vi "Teleop.vi"(10 "Match Info":T1={"Autonomous Elapsed Seconds"=0.0, "TeleOp Elapsed Seconds"=0.0, "Disabled Elapsed Seconds"=0.0, "Visited Autonomous"=FALSE, "Visited TeleOp"=FALSE, "Visited Disabled"=FALSE, "Autonomous Settings"={"Autonomous Style"=enum."Independent", "VI Refnum"=refnum}}, 11 "Call Context":T2) -> ()   [LabVIEW 2023]
doc: "This VI is called for each TeleOp packet received from the DS where the robot is not disabled. It is often used to read from the joysticks and update I/O or to update setpoints for timed control loops. It should complete and return within 20 milliseconds or it may miss DS packets."
uses:
  <vilib>/Rock Robotics/WPI/DriverStation/WPI_DriverStationDerivedRobotMode.ctl
  <vilib>/Rock Robotics/WPI/DriverStation/WPI_DriverStationMatch Info.ctl
  <vilib>/Rock Robotics/Network Tables/NT Read Boolean.vi
  <vilib>/Rock Robotics/WPI/Utilities/WPI_GetSetVariantRefNum.vi
  variavelVelocidades.vi
  <vilib>/Rock Robotics/Network Tables/NT Read Number.vi
  <vilib>/Rock Robotics/WPI/RobotDrive/WPI_RobotDriveArcadeDrive_Standard(NoSaturation).vi
  <vilib>/Rock Robotics/Network Tables/NT Write Boolean.vi
panel:
  out "botaoAtivado?":bool
  out "Sample Slider 0":dbl(slide) scale=0.0..5.0
  out "Sample Boolean 1":bool
  out "Sample Boolean 0":bool
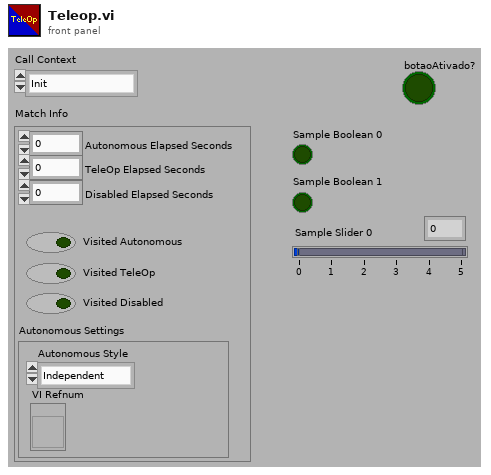
[diagram p1: front panel]
types:
  T1 = typedef "WPI_DriverStationMatch Info.ctl" = cluster{"Autonomous Elapsed Seconds":dbl, "TeleOp Elapsed Seconds":dbl, "Disabled Elapsed Seconds":dbl, "Visited Autonomous":bool, "Visited TeleOp":bool, "Visited Disabled":bool, "Autonomous Settings":cluster{"Autonomous Style":enum16{"Iterative", "Independent"}, "VI Refnum":refnum<vi>}}
  T2 = typedef "WPI_DriverStationDerivedRobotMode.ctl" = enum16{"Init", "Execute", "Stop"}
  T3 = typedef "WPI_JoystickDevRef.ctl" = cluster{"Device":T4}
  T4 = typedef "WPI_JoystickDeviceEnum.ctl" = enum16{"USB 0", "USB 1", "USB 2", "USB 3", "USB 4", "USB 5"}
  T5 = typedef "WPI_RobotDriveDevRef.ctl" = cluster{"DevStatus":errorcluster, "Motors[]":T6[], "Square Inputs":bool, "Max Output":dbl}
  T6 = typedef "WPI_MotorControlDeviceRef.ctl" = cluster{"DeviceStatus":errorcluster, "Type":T7, "PWM":cluster{"PWM Channel":T8, "DeadBand":T9}, "CAN":cluster{"Device Number":u8, "SetOutput VI Ref":variant, "GetOutput VI Ref":variant, "Enable VI Ref":variant, "Disable VI Ref":variant, "Data":variant}, "Invert":bool, "DIO PWM":cluster{"PWM \"Enable\" Channel":T8, "DIOChannel":T10, "PWM Rate":dbl}}
  T7 = typedef "WPI_MotorControlType.ctl" = enum16{"PWM", "CAN", "DIO PWM"}
  T8 = typedef "FPGA_DIOPWMChannel.ctl" = enum8{"PWM 0", "PWM 1", "PWM 2", "PWM 3", "PWM 4", "PWM 5", "PWM 6", "PWM 7", "PWM 8", "PWM 9", "PWM MXP 0", "PWM MXP 1", "PWM MXP 2", "PWM MXP 3", "PWM MXP 4", "PWM MXP 5", "PWM MXP 6", "PWM MXP 7", "PWM MXP 8", "PWM MXP 9", "Invalid"}
  T9 = typedef "WPI_PWMDeadband.ctl" = cluster{"Name":string, "maxPositivePwm":i32, "minPositivePwm":i32, "centerPwm":i32, "maxNegativePwm":i32, "minNegativePwm":i32, "angularRange":u16}
  T10 = typedef "FPGA_DIOChannel.ctl" = enum8{"DIO 0", "DIO 1", "DIO 2", "DIO 3", "DIO 4", "DIO 5", "DIO 6", "DIO 7", "DIO 8", "DIO 9", "DIO MXP 0", "DIO MXP 1", "DIO MXP 2", "DIO MXP 3", "DIO MXP 4", "DIO MXP 5", "DIO MXP 6", "DIO MXP 7", "DIO MXP 8", "DIO MXP 9", "DIO MXP 10", "DIO MXP 11", "DIO MXP 12", "DIO MXP 13", "DIO MXP 14", "DIO MXP 15", "SPI Port CS1", "SPI Port CS2", "SPI Port CS3", "SPI Port MISO", "SPI Port MOSI", "Invalid"}
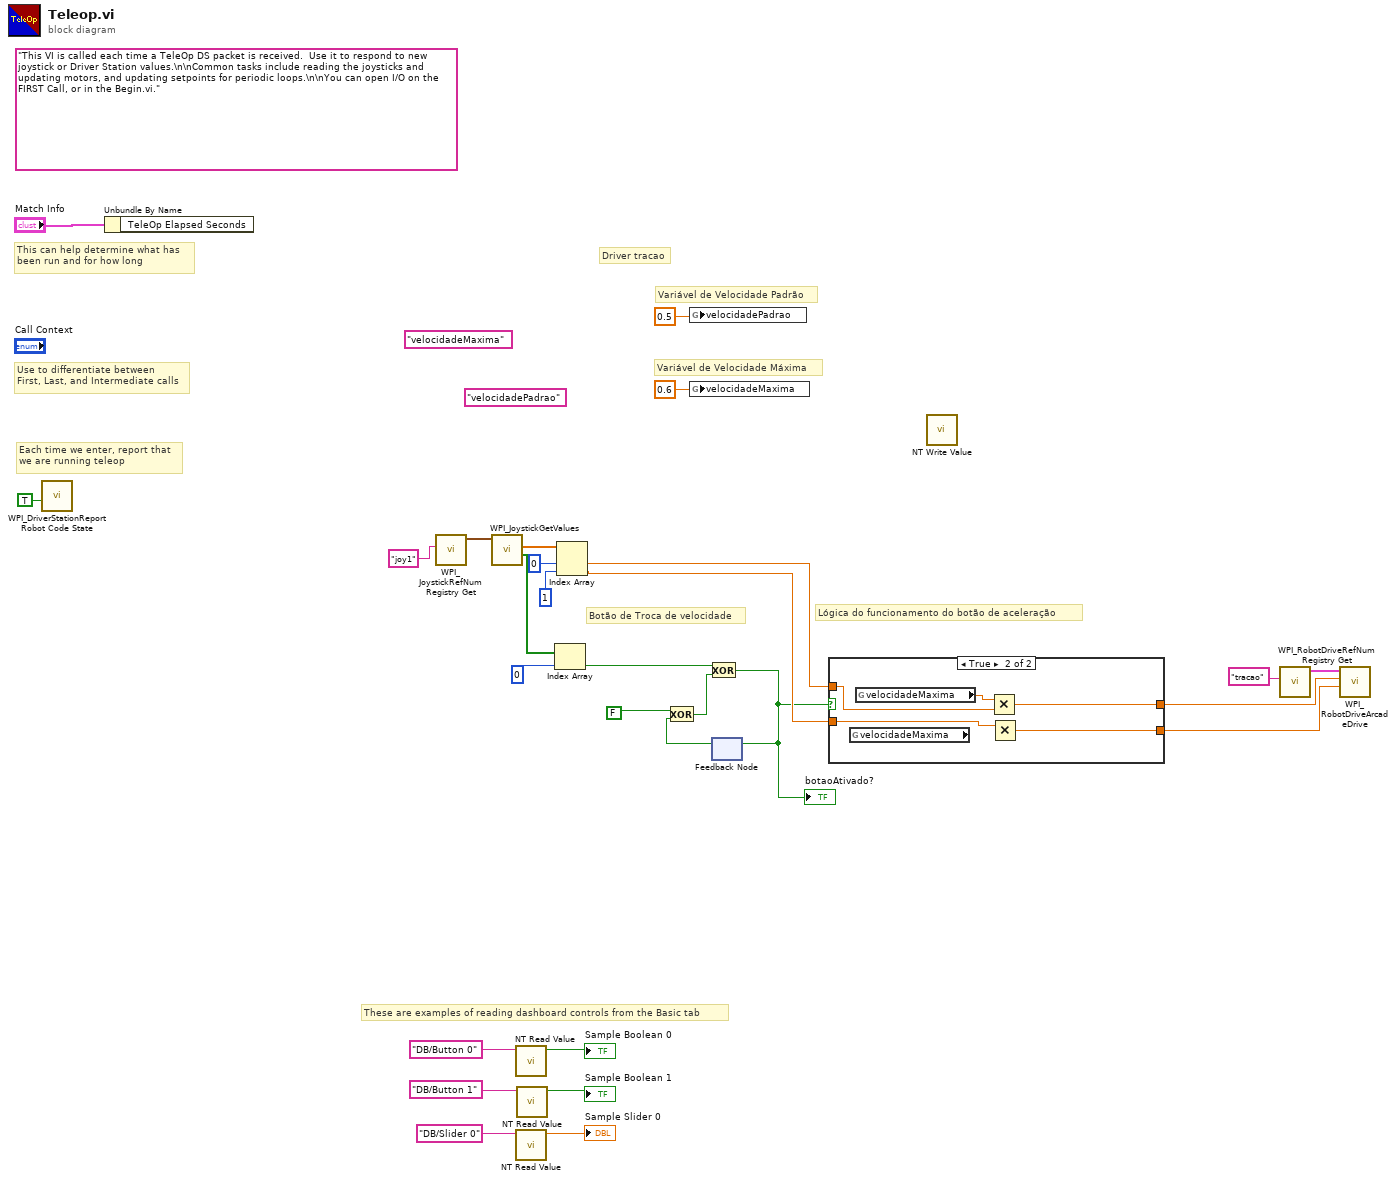
[diagram p0: block diagram]
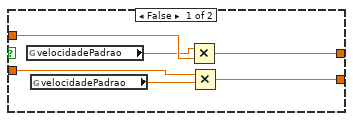
[diagram p2: hidden frame]
diagram:
  (unwired) "velocidadePadrao"
  (unwired) "velocidadeMaxima"
  (unwired) "This VI is called each time a TeleOp DS packet is received.  Use it to respond to new joystick or Driver Station values.\n\nCommon tasks include reading the joysticks and updating motors, and updating setpoints for periodic loops.\n\nYou can open I/O on the FIRST Call, or in the Begin.vi."
  # "Variável de Velocidade Máxima"
  # "Variável de Velocidade Padrão"
  # "Botão de Troca de velocidade"
  # "Lógica do funcionamento do botão de aceleração"
  # "These are examples of reading dashboard controls from the Basic tab"
  # "Each time we enter, report that\nwe are running teleop"
  # "Use to differentiate between\nFirst, Last, and Intermediate calls"
  # "This can help determine what has\nbeen run and for how long"
  # "Driver tracao"
  n1 = call <vilib>:"WPI_DriverStationReport Robot Code State.vi"("TeleOp"=TRUE ("Autonomous")) -> ()  [unwired: 10 in, 1 out]
  n2 = Unbundle By Name("Match Info") -> ()  [unwired: 1 out]
  n3 = call <vilib>:"WPI_JoystickRefNum Registry Get.vi"("refnum name"="joy1") -> ("JoystickDevRef"=w20:T3)  [unwired: 9 in, 1 out]
  n4 = call <vilib>:"WPI_JoystickGetValues.vi"("JoystickDevRef"=w20) -> ("Buttons"=w14:bool[], "Axes"=w18:dbl[])  [unwired: 6 in, 3 out]
  n5 = call-poly <vilib>:"NT Read Value.vi"("name"="DB/Button 0" ("refnum name")) -> ("value"=→"Sample Boolean 0":bool)  [unwired: 8 in, 2 out]
  n6 = call-poly <vilib>:"NT Read Value.vi"("name"="DB/Slider 0" ("refnum name")) -> ("value"=→"Sample Slider 0":dbl)  [unwired: 8 in, 2 out]
  n7 = call-poly <vilib>:"NT Read Value.vi"("name"="DB/Button 1" ("refnum name")) -> ("value"=→"Sample Boolean 1":bool)  [unwired: 8 in, 2 out]
  n8 = Index Array(array=w14, index=0) -> (element=w12:bool)
  n9 = Index Array(array=w18, index #1=0 ("index"), index #2=1 ("index")) -> (element #1=w6:dbl, element #2=w5:dbl)
  n10 = global write "variavelVelocidades.vi" "velocidadePadrao"(0.5 ("velocidadePadrao")) -> ()
  n11 = global write "variavelVelocidades.vi" "velocidadeMaxima"(0.6 ("velocidadeMaxima")) -> ()
  n12 = feedback #1() -> (w10:bool)  [unwired: 1 in]
  n13 = Exclusive Or(1:w10, 2:FALSE ("x")) -> (0:w11:bool)
  n14 = Exclusive Or(1:w11, 2:w12) -> (0:w4:bool)
  "botaoAtivado?" <- w4
  n15 = feedback-in #1(w4) -> ()
  n16 = case shown="True" w4 {
    tunnel: [w34 w39] -> w8
    tunnel: [w33 w38] -> w7
    tunnel: w6 -> [w32 w37]
    tunnel: w5 -> [w31 w36]
    frame False {
      n17 = global read "variavelVelocidades.vi" "velocidadePadrao"() -> (w30:dbl)
      n18 = global read "variavelVelocidades.vi" "velocidadePadrao"() -> (w29:dbl)
      n19 = Multiply(x=w30, y=w32) -> (x*y=w34:dbl)
      n20 = Multiply(x=w31, y=w29) -> (x*y=w33:dbl)
    }
    frame True {
      n21 = global read "variavelVelocidades.vi" "velocidadeMaxima"() -> ()  [unwired: 1 out]
      n22 = global read "variavelVelocidades.vi" "velocidadeMaxima"() -> (w35:dbl)
      n23 = Multiply(x=w35, y=w37) -> (x*y=w39:dbl)
      n24 = Multiply(x=w36) -> (x*y=w38:dbl)  [unwired: 1 in]
    }
  }
  n25 = call-poly <vilib>:"NT Write Value.vi"() -> ()  [unwired: 11 in, 1 out]
  n26 = call <vilib>:"WPI_RobotDriveRefNum Registry Get.vi"("refnum name"="tracao") -> ("RobotDriveDevRef"=w15:T5)  [unwired: 9 in, 1 out]
  n27 = call-poly <vilib>:"WPI_RobotDriveArcadeDrive.vi"("Y axis value"=w7, "X axis value"=w8, "RobotDriveDevRef"=w15) -> ()  [unwired: 6 in, 3 out]
